vi "Execute Query.vi"(8 "error in (no error)":errorcluster, 9 "Parâmetros":T1[](array[typedef]), 10 "SQL query":string, 11 "Connection in":T2) -> (0 "error out":errorcluster, 1 "Query Time":dbl, 2 "data":string[][](array[string]), 3 "Connection out":T2, 4 "Sem dados?":bool)   [LabVIEW 2020, in "PostgreSQL Driver.lvlib"]
uses:
  PostgreSQL Driver.lvlib
  <vilib>/addons/database/Connection.llb/Conn ObjectReference.ctl
  <vilib>/addons/database/Connection.llb/Conn Execute.vi
  <vilib>/addons/database/Recordset.llb/Rec Fetch Recordset Data (R).vi
  <vilib>/addons/database/Recordset.llb/Rec Destroy - Connection.vi
  <vilib>/addons/database/NI_Database_API.lvlib
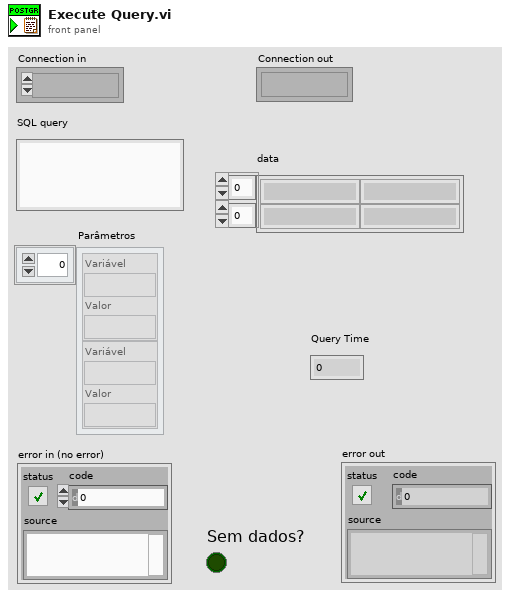
[diagram p1: front panel]
types:
  T1 = typedef "PostgreSQL Driver.lvlib/Parâmetros Execute Query.ctl" = cluster{"Variável":string, "Valor":string}
  T2 = typedef "NI_Database_API.lvlib/Conn ObjectReference.ctl" = refnum<k1>
  T3 = typedef "NI_Database_API.lvlib/Rec ObjectReference.ctl" = refnum<k1>
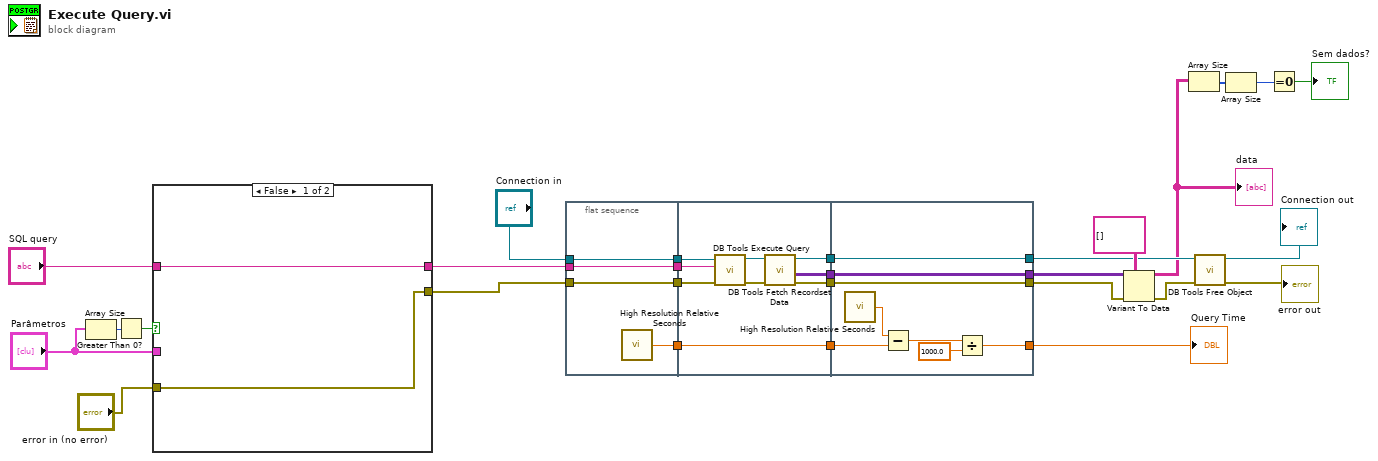
[diagram p0: block diagram]
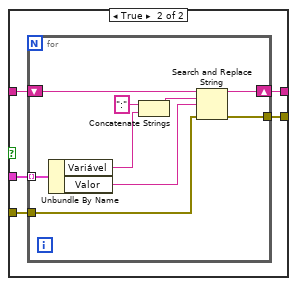
[diagram p2: hidden frame]
diagram:
  n1 = Array Size(array="Parâmetros") -> (size(s)=w10:i32)
  n2 = Greater Than 0?(x=w10) -> (x > 0?=w11:bool)
  n3 = case shown="False" w11 {
    tunnel: "Parâmetros" -> [_ w35]
    tunnel: "SQL query" -> [w30 w34]
    tunnel: [w30 w33] -> w8
    tunnel: "error in (no error)" -> [w29 w32]
    tunnel: [w29 w31] -> w6
    frame False {
    }
    frame True {
      n4 = for {
        tunnel: w35 -> [w44] mode=indexing
        shift-right: [w42] -> w33
        shift-left: w34 -> [w43]
        tunnel: w32 -> [w37]
        tunnel: [w36] -> w31
        n5 = Unbundle By Name(w44) -> ("Variável"=w39:string, "Valor"=w41:string)
        n6 = Concatenate Strings(":" ("string"), w39) -> (w40:string)
        n7 = Search and Replace String(input string=w43, search string=w40, replace string=w41, error in=w37) -> (result string=w42:string, error out=w36:errorcluster)  [unwired: 4 in, 2 out]
      }
    }
  }
  n8 = flat-sequence {
    tunnel: w8 -> [w47]
    tunnel: "Connection in" -> [w48]
    tunnel: [w48] -> w28
    tunnel: [w47] -> w27
    tunnel: [w46] -> w26
    tunnel: w6 -> [w45]
    tunnel: [w45] -> w5
    tunnel: w28 -> [w54]
    tunnel: w27 -> [w51]
    tunnel: [w55] -> w25
    tunnel: [w53] -> w24
    tunnel: [w52] -> w23
    tunnel: w26 -> [w50]
    tunnel: [w50] -> w22
    tunnel: w5 -> [w49]
    tunnel: [w63] -> w19
    tunnel: [w64] -> w17
    tunnel: [w65] -> w13
    tunnel: w25 -> [w65]
    tunnel: w24 -> [w64]
    tunnel: w23 -> [w63]
    tunnel: w22 -> [w61]
    tunnel: [w58] -> w21
    frame #0 {
      n9 = call <vilib>:"High Resolution Relative Seconds.vi"() -> ("relative seconds"=w46:dbl)
    }
    frame #1 {
      n10 = call-poly <vilib>:"DB Tools Execute Query.vi"("error in (no error)"=w49, "SQL query"=w51, "connection reference"=w54) -> ("error out"=w57:errorcluster, "recordset reference"=w56:T3)  [unwired: 5 in]
      n11 = call-poly <vilib>:"DB Tools Fetch Recordset Data.vi"("error in (no error)"=w57, "recordset reference"=w56) -> ("error out"=w52:errorcluster, "recordset data"=w53:variant[][], "recordset reference out"=w55:T3)  [unwired: 3 in]
    }
    frame #2 {
      n12 = call <vilib>:"High Resolution Relative Seconds.vi"() -> ("relative seconds"=w62:dbl)
      n13 = Subtract(x=w62, y=w61) -> (x-y=w60:dbl)
      n14 = Divide(x=w60, y=1000.0) -> (x/y=w58:dbl)
    }
  }
  n15 = Variant To Data(error in=w19, type=string[][] [], Variant=w17) -> (data=w4:string[][], error out=w20:errorcluster)
  "data" <- w4
  n16 = Array Size(array=w4) -> (size(s)=w3:i32[])
  n17 = call-poly <vilib>:"DB Tools Free Object.vi"("error in (no error)"=w20, "recordset reference"=w13) -> ("error out"=→"error out":errorcluster, "connection reference"=→"Connection out":T2)  [unwired: 8 in]
  n18 = Array Size(array=w3) -> (size(s)=w2:i32)
  n19 = Equal To 0?(x=w2) -> (x = 0?=→"Sem dados?":bool)
  "Query Time" <- w21
